vi "Show Temp Rise values.vi"(7 "Panel":u64, 8 "MaxTRise":dbl=150.0, 9 "(SIG) in":T1, 10 "Temp Strt in":cluster{"TL":dbl, "TN":dbl}, 11 "T Rise":cluster{dbl, dbl}) -> (2 "Invalid T Rise":bool)   [LabVIEW 2017]
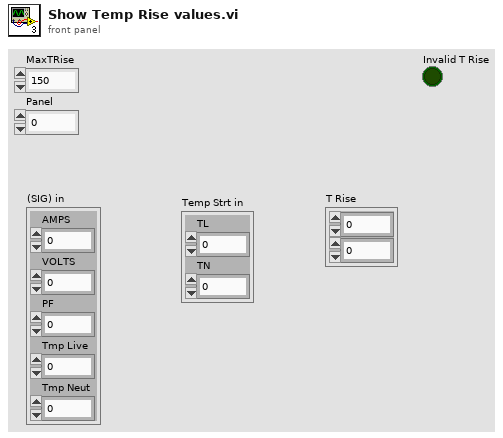
[diagram p1: front panel]
types:
  T1 = cluster{"AMPS":dbl, "VOLTS":dbl, "PF":dbl, "Tmp Live":dbl, "Tmp Neut":dbl}
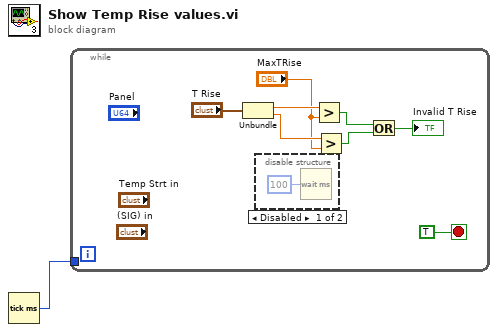
[diagram p0: block diagram]
diagram:
  n1 = Tick Count (ms)() -> (millisecond timer value=w1:u32)
  n2 = while {
    tunnel: w1 -> [_]
    stop <- TRUE stop-if-true
    n3 = Unbundle("T Rise") -> (w7:dbl, w6:dbl)
    n4 = disable-structure shown="Disabled" {
      frame Disabled {
        n5 = Wait (ms)(milliseconds to wait=u32 100) -> ()  [unwired: 1 out]
      }
      frame Enabled {
      }
    }
    n6 = Greater?(x=w7, y="MaxTRise") -> (0:w3:bool)
    n7 = Greater?(x=w6, y="MaxTRise") -> (0:w4:bool)
    n8 = Or(x=w3, y=w4) -> (x .or. y?=→"Invalid T Rise":bool)
  }
